vi "read TDMS photometry waveform file.vi"() -> ()   [LabVIEW 2013]
panel:
  out "Signals":dynamicdata(graph)
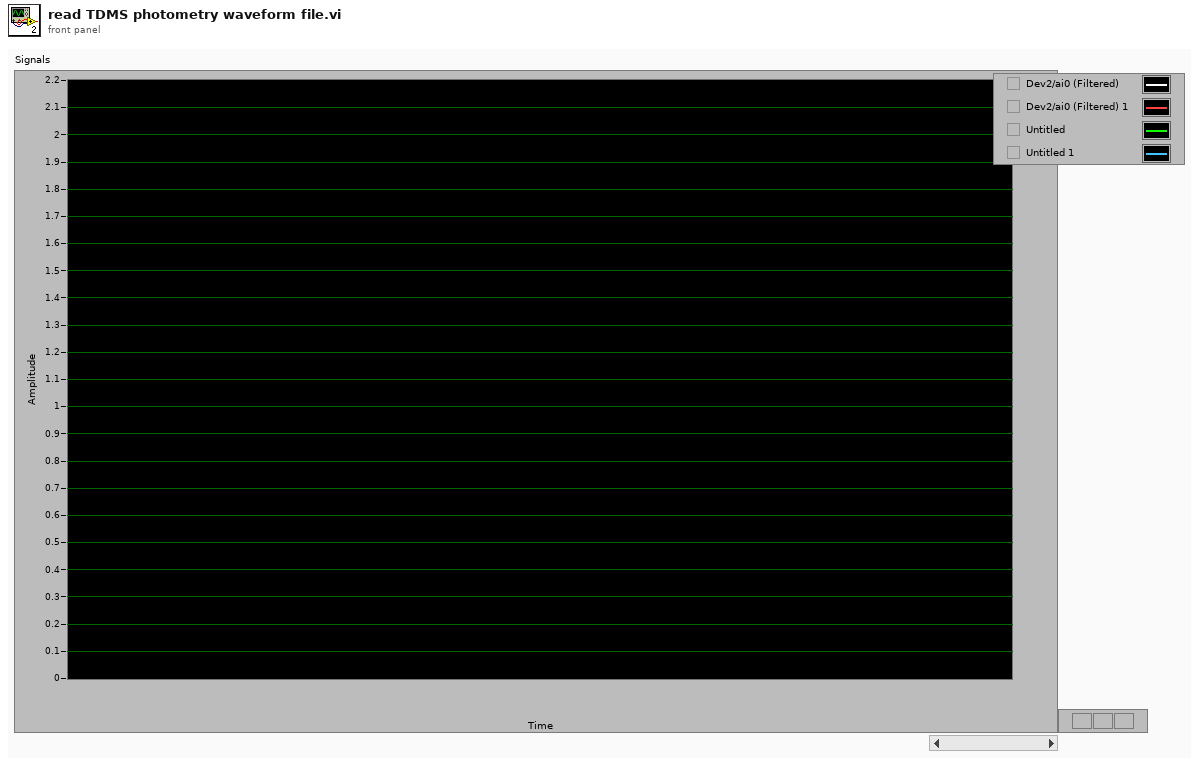
[diagram p1: front panel]
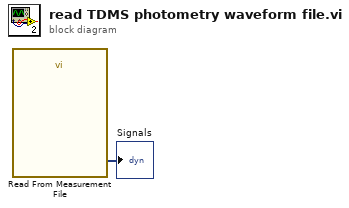
[diagram p0: block diagram]
diagram:
  n1 = call "Read From Measurement File"() -> ("Signals"=→"Signals":dynamicdata)  [unwired: 6 in, 5 out]
